vi "Save.vi"(8 "czêstotliwoœæ":dbl[](array[numeric]), 9 "Wartosci na wyjsciu":dbl[](array[numeric]), 11 "Wartosci na wejsciu":dbl[](array[numeric])) -> ()   [LabVIEW 2018]
doc: "Zapisuje wyniki pomiarów do pliku."
uses:
  <vilib>/Utility/file.llb/Write Delimited Spreadsheet (string).vi
panel:
  out "error out 3":errorcluster
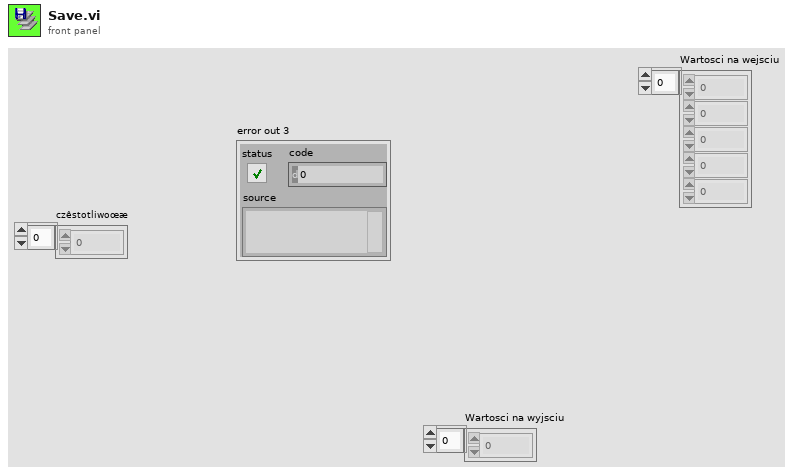
[diagram p1: front panel]
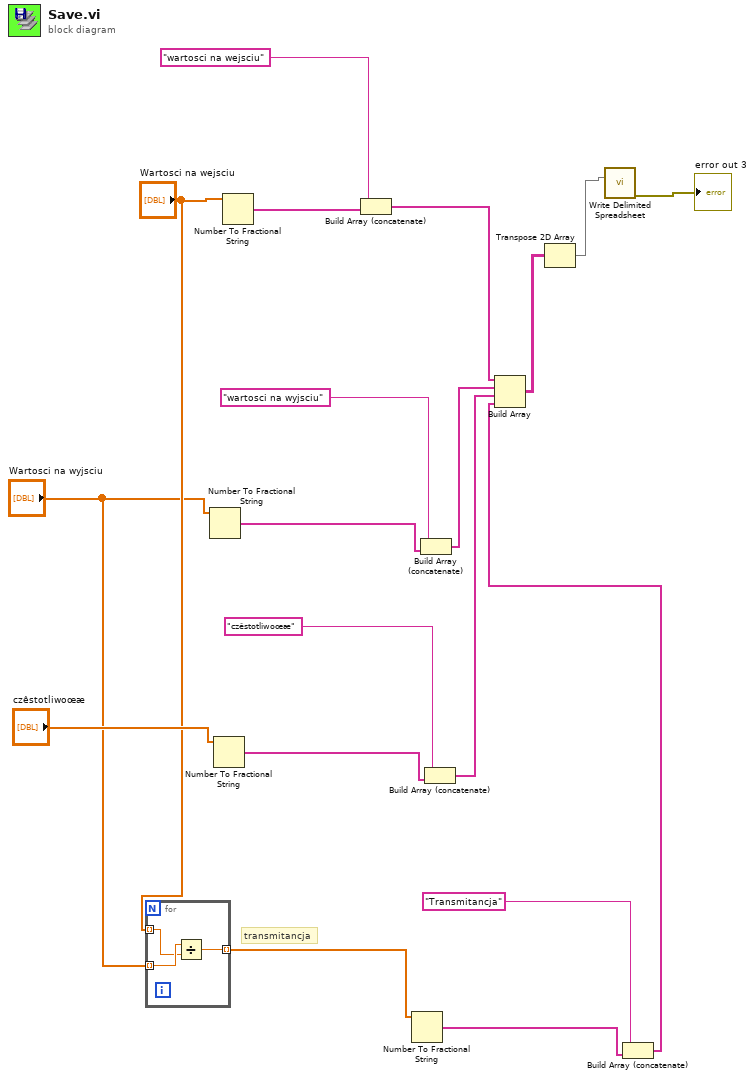
[diagram p0: block diagram]
diagram:
  # "transmitancja"
  n1 = for {
    tunnel: "Wartosci na wejsciu" -> [w21] mode=indexing
    tunnel: "Wartosci na wyjsciu" -> [w22] mode=indexing
    tunnel: [w20] -> w2 mode=indexing
    n2 = Divide(x=w22, y=w21) -> (x/y=w20:dbl)
  }
  n3 = Number To Fractional String(number="Wartosci na wyjsciu") -> (F-format string=w11:string[])  [unwired: 3 in]
  n4 = Number To Fractional String(number="czêstotliwoœæ") -> (F-format string=w8:string[])  [unwired: 3 in]
  n5 = Number To Fractional String(number="Wartosci na wejsciu") -> (F-format string=w12:string[])  [unwired: 3 in]
  n6 = Build Array (concatenate)("wartosci na wejsciu", w12) -> (w15:string[])
  n7 = Number To Fractional String(number=w2) -> (F-format string=w3:string[])  [unwired: 3 in]
  n8 = Build Array (concatenate)("wartosci na wyjsciu", w11) -> (w16:string[])
  n9 = Build Array (concatenate)("czêstotliwoœæ", w8) -> (w7:string[])
  n10 = Build Array (concatenate)("Transmitancja", w3) -> (w1:string[])
  n11 = Build Array(w15, w16, w7, w1) -> (w14:string[][])
  n12 = Transpose 2D Array(2D array=w14) -> (transposed array=w13:string[][])
  n13 = call-poly <vilib>:"Write Delimited Spreadsheet.vi"("2D data"=w13) -> ("error out"=→"error out 3":errorcluster)  [unwired: 13 in, 1 out]
